vi "BT_to_neon.vi"() -> ()   [LabVIEW 2016]
uses:
  Typedef/Type_of_message_to_MCU.ctl
  Typedef/MCU_addresses.ctl
  Typedef/Serial_config_cluster.ctl
  <vilib>/Instr/_visa.llb/VISA Configure Serial Port (Instr).vi
panel:
  out "error out":errorcluster
  in  "Cluster 2":T1={"Termination Character"=10, "End Read on"=TRUE, "VISA resource name"="COM1", "baud rate"=9600, "data bits"=8, "parity"=enum."None", "stop bits"=10, "flow control"=0, "XON"=enum."DC1", "XOFF"=enum."DC3", "End Write on"=FALSE} {"Termination Character" format="%.0x"; "flow control" items=["None"=0, "XON/XOFF"=1, "RTS/CTS"=2, "DTR/DSR"=4]; "data bits" min=5 max=8 step=1; "stop bits" items=["1.0"=10, "1.5"=15, "2.0"=20]; "baud rate" items=["75"=75, "110"=110, "134"=134, "150"=150, "300"=300, "600"=600, "1200"=1200, "1800"=1800, "2400"=2400, "4800"=4800, "7200"=7200, "9600"=9600, "14400"=14400, "19200"=19200, "28800"=28800, "38400"=38400, "56000"=56000, "57600"=57600, "115200"=115200, "128000"=128000, "230400"=230400]}
  in  "Stop\n 2":bool
  in  "Read Count 2":u32=1000
  out "String 2":string
  out "Extracted Numbers 2":dbl[](array[numeric]) format="%#.6g"
  in  "Save 2":bool=TRUE
  out "Array 2":dbl[](array[numeric])
  out "Waveform Chart 2":dynamicdata(graph)
  in  "index 6":i32
  in  "index 5":i32
  in  "index 4":i32
  in  "y 2":dbl=15.0 format="%#_13g"
  in  "FIltering 2":bool
  out "Byte array has been sent 2":u8[](array[numeric])
  in  "MCU Address to be sent 2":T2
  in  "Payload  Byte to be sent 2":u8[](array[numeric])
  in  "Types of Data 2":T3
  in  "Read 2":bool=TRUE
  out "Bytes at Serial Port 2":u32
  out "error out 3":errorcluster
  in  "MAIN STOP 2":bool
  out "MAIN STOP OUT 2":bool
  in  "sEND":bool
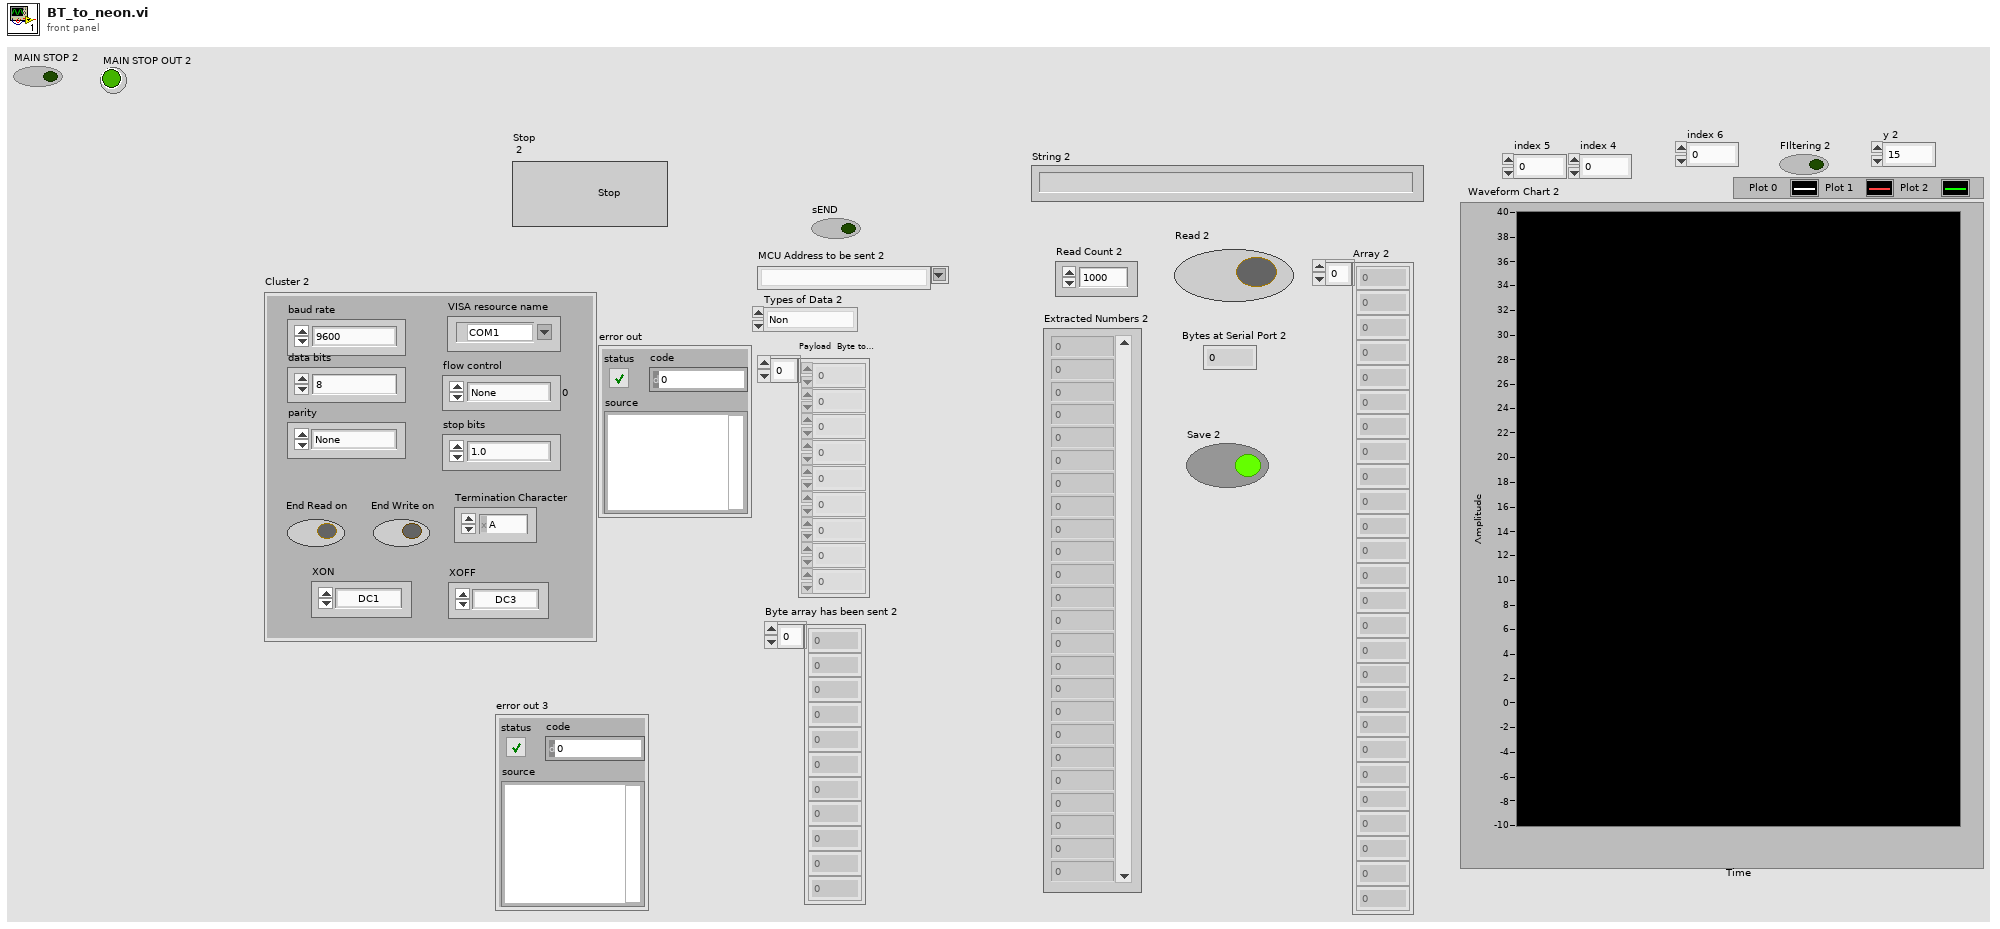
[diagram p1: front panel]
types:
  T1 = typedef "Serial_config_cluster.ctl" = cluster{"Termination Character":u8, "End Read on":bool, "VISA resource name":refnum<visa-resource-name>, "baud rate":u32, "data bits":u16, "parity":enum16{"None", "Odd", "Even", "Mark", "Space"}, "stop bits":u16, "flow control":u16, "XON":enum16{"NUL", "SOH", "STX", "ETX", "EOT", "ENQ", "ACK", "BEL", "BS", "HT", "LF", "VT", "FF", "CR", "SO", "SI", "DLE", "DC1", "DC2", "DC3", "DC4", "NAK", "SYN", "ETB", "CAN", "EM", "SUB", "ESC", "FS", "GS", "RS", "US", "SP", "!", "\"", "#", "$", "%", "&", "'", "(", ")", "*", "+", ",", "- (-)", ".", "/", "0", "1", "2", "3", "4", "5", "6", "7", "8", "9", ":", ";", "<", "=", ">", "?", "@", "A", "B", "C", "D", "E", "F", "G", "H", "I", "J", "K", "L", "M", "N", "O", "P", "Q", "R", "S", "T", "U", "V", "W", "X", "Y", "Z", "[", "\\", "]", "^", "_", "`", "a", "b", "c", "d", "e", "f", "g", "h", "i", "j", "k", "l", "m", "n", "o", "p", "q", "r", "s", "t", "u", "v", "w", "x", "y", "z", "{", "|", "}", "~"}, "XOFF":enum16{"NUL", "SOH", "STX", "ETX", "EOT", "ENQ", "ACK", "BEL", "BS", "HT", "LF", "VT", "FF", "CR", "SO", "SI", "DLE", "DC1", "DC2", "DC3", "DC4", "NAK", "SYN", "ETB", "CAN", "EM", "SUB", "ESC", "FS", "GS", "RS", "US", "SP", "!", "\"", "#", "$", "%", "&", "'", "(", ")", "*", "+", ",", "- (-)", ".", "/", "0", "1", "2", "3", "4", "5", "6", "7", "8", "9", ":", ";", "<", "=", ">", "?", "@", "A", "B", "C", "D", "E", "F", "G", "H", "I", "J", "K", "L", "M", "N", "O", "P", "Q", "R", "S", "T", "U", "V", "W", "X", "Y", "Z", "[", "\\", "]", "^", "_", "`", "a", "b", "c", "d", "e", "f", "g", "h", "i", "j", "k", "l", "m", "n", "o", "p", "q", "r", "s", "t", "u", "v", "w", "x", "y", "z", "{", "|", "}", "~"}, "End Write on":bool}
  T2 = typedef "MCU_addresses.ctl" = string
  T3 = typedef "Type_of_message_to_MCU.ctl" = enum16{"Non", "Alarm", "Error", "Time and Date", "Status", "Request", "Command"}
  T4 = enum16{"NUL", "SOH", "STX", "ETX", "EOT", "ENQ", "ACK", "BEL", "BS", "HT", "LF", "VT", "FF", "CR", "SO", "SI", "DLE", "DC1", "DC2", "DC3", "DC4", "NAK", "SYN", "ETB", "CAN", "EM", "SUB", "ESC", "FS", "GS", "RS", "US", "SP", "!", "\"", "#", "$", "%", "&", "'", "(", ")", "*", "+", ",", "- (-)", ".", "/", "0", "1", "2", "3", "4", "5", "6", "7", "8", "9", ":", ";", "<", "=", ">", "?", "@", "A", "B", "C", "D", "E", "F", "G", "H", "I", "J", "K", "L", "M", "N", "O", "P", "Q", "R", "S", "T", "U", "V", "W", "X", "Y", "Z", "[", "\\", "]", "^", "_", "`", "a", "b", "c", "d", "e", "f", "g", "h", "i", "j", "k", "l", "m", "n", "o", "p", "q", "r", "s", "t", "u", "v", "w", "x", "y", "z", "{", "|", "}", "~"}
  T5 = typedef "Message_info.ctl" = enum16{"Non", "Earthquake", "Fire", "Lost Power", "New", "Restarted"}
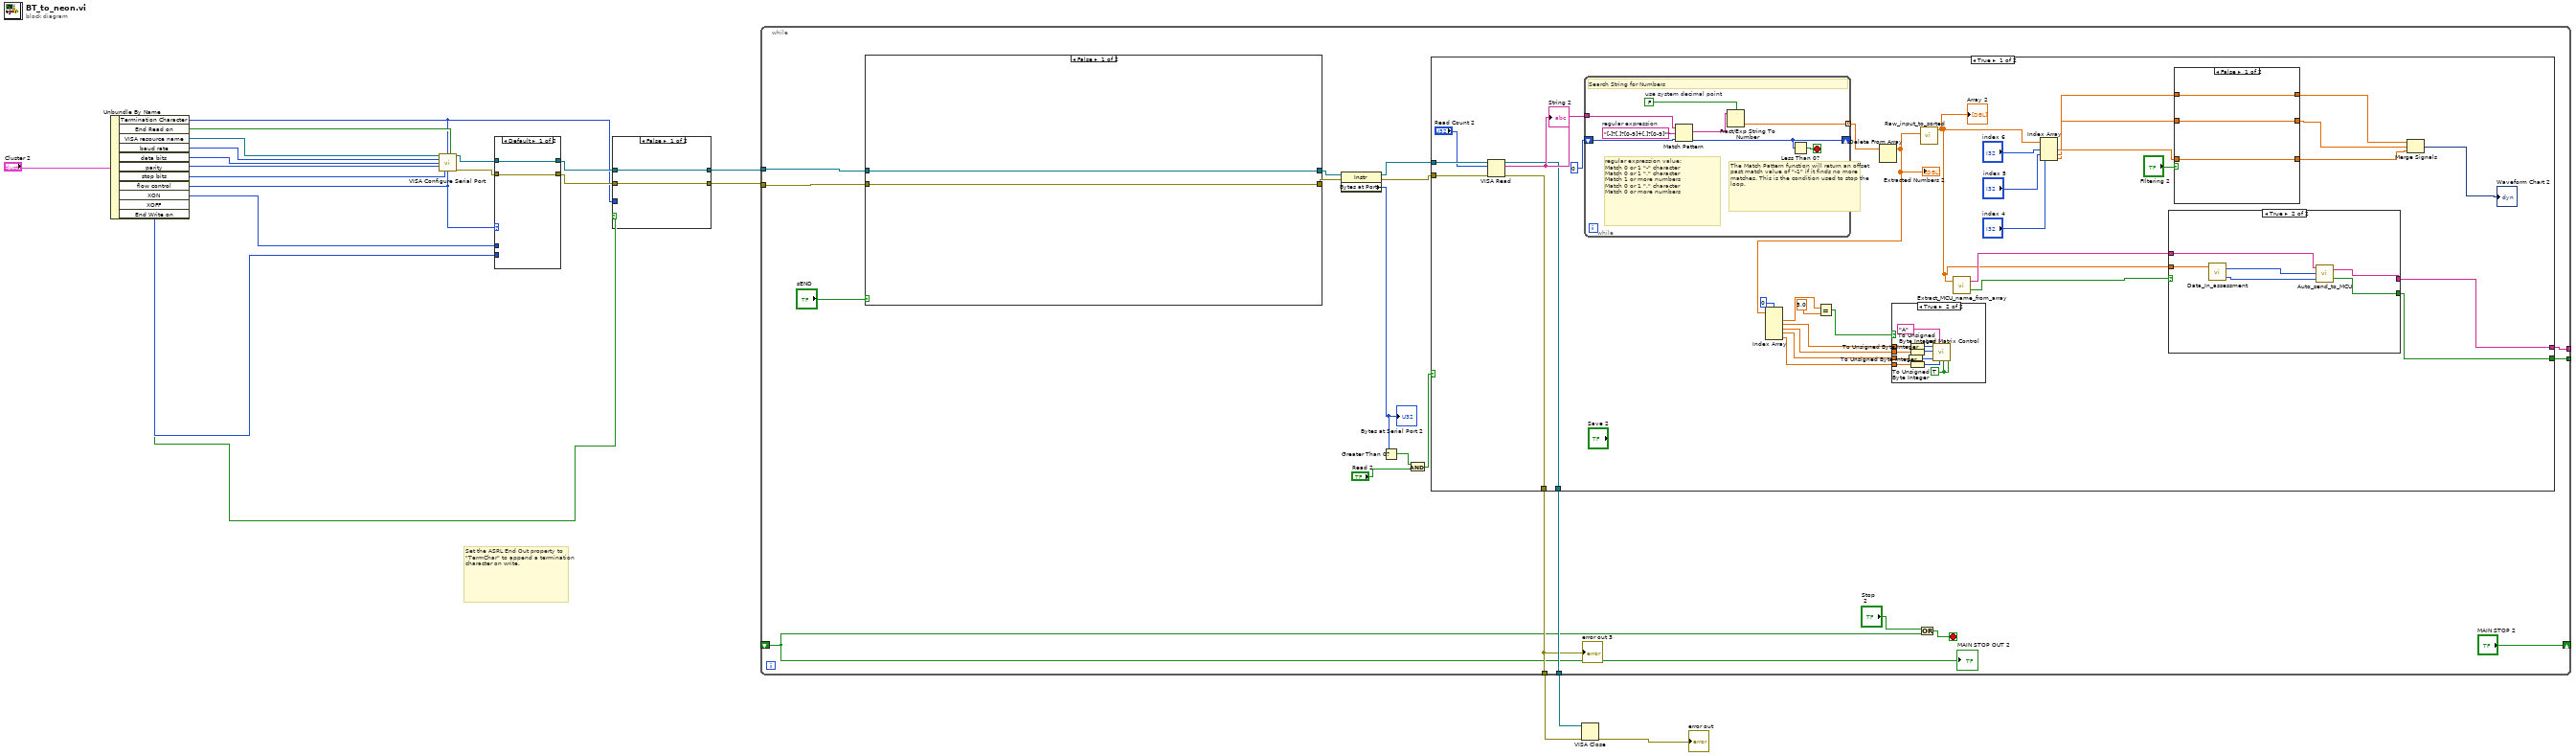
[diagram p0: block diagram]
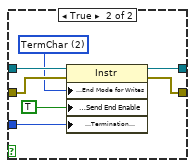
[diagram p2: hidden frame]
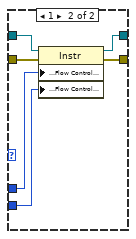
[diagram p3: hidden frame]
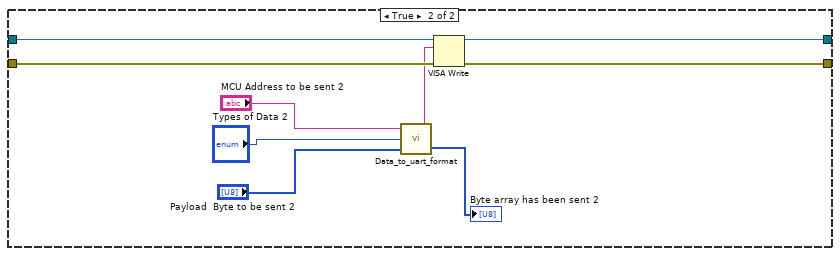
[diagram p4: hidden frame]
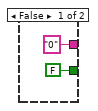
[diagram p6: hidden frame]
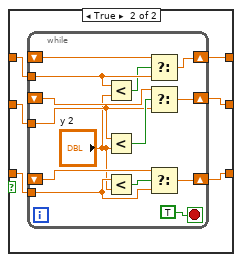
[diagram p7: hidden frame]
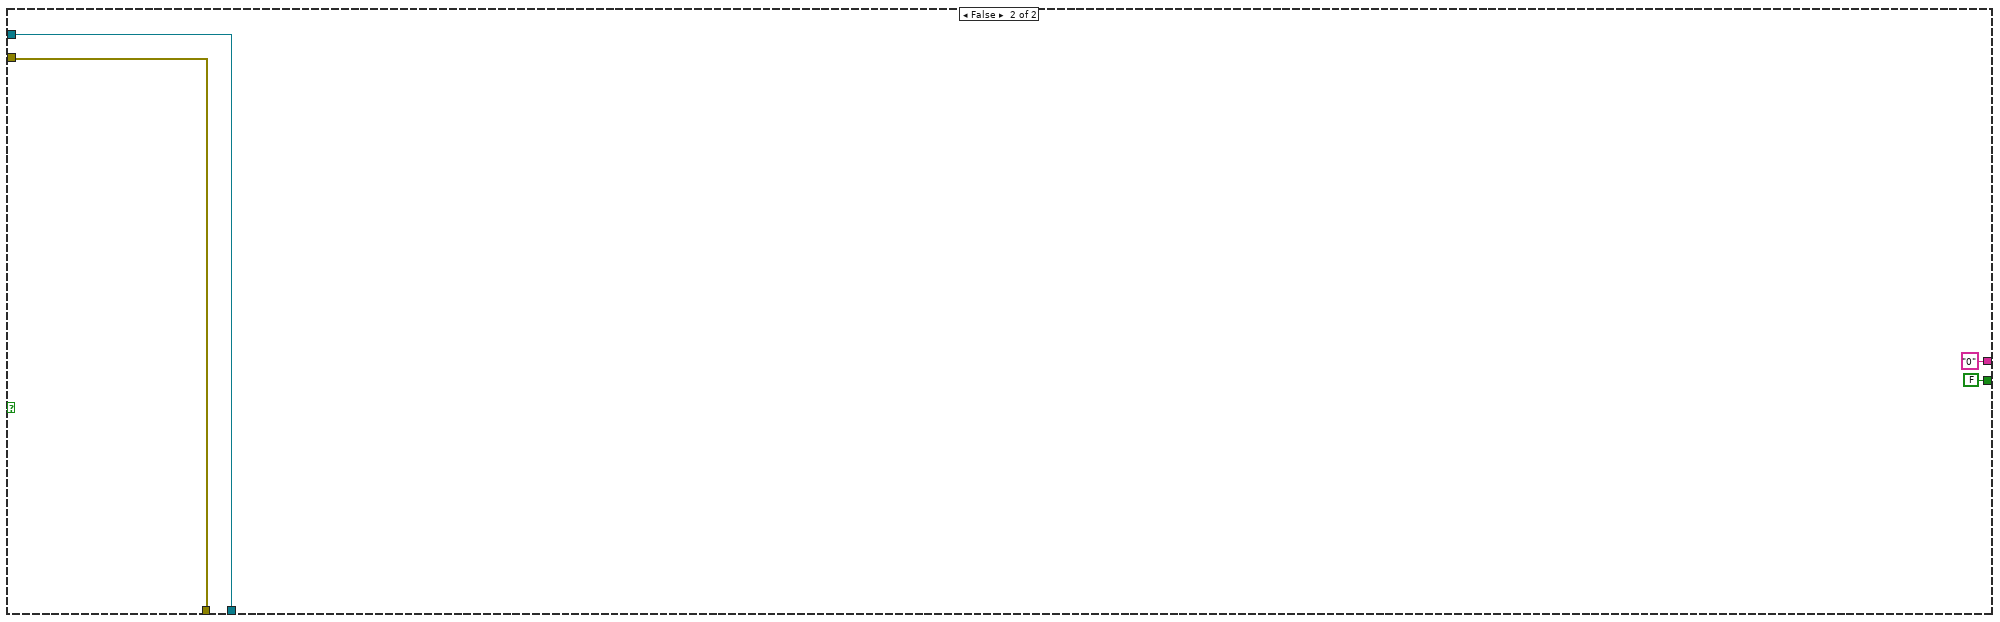
[diagram p8: hidden frame]
diagram:
  # "Set the ASRL End Out property to \"TermChar\" to append a termination character on write."
  n1 = Unbundle By Name("Cluster 2") -> ("Termination Character"=w6:u8, "End Read on"=w15:bool, "VISA resource name"=w16:refnum<visa-resource-name>, "baud rate"=w14:u32, "data bits"=w13:u16, "parity"=w12:enum16{"None", "Odd", "Even", "Mark", "Space"}, "stop bits"=w11:u16, "flow control"=w10:u16, "XON"=w9:T4, "XOFF"=w8:T4, "End Write on"=w7:bool)
  n2 = call-poly "VISA Configure Serial Port"("VISA resource name"=w16, "termination char\n(0xA = '\\n' = LF)"=w6, "Enable Termination\nChar (T)"=w15, "baud rate (9600)"=w14, "data bits (8)"=w13, "parity (0:none)"=w12, "stop bits (10: 1 bit)"=w11, "flow control (0:none)"=w10) -> ("VISA resource name out"=w19:refnum<visa-resource-name>, "error out"=w18:errorcluster)  [unwired: 2 in, 4 out]
  n3 = case shown="Default" w10 {
    tunnel: [w22 w29] -> w20
    tunnel: [w23 w28] -> w21
    tunnel: w18 -> [w22 w27]
    tunnel: w19 -> [w23 w26]
    tunnel: w9 -> [_ w25]
    tunnel: w8 -> [_ w24]
    frame Default {
    }
    frame 1 {
      n4 = property class="Instr"(reference=w26, error in=w27, "Serial Settings:Flow Control XON Character"=w25, "Serial Settings:Flow Control XOFF Character"=w24) -> (reference out=w28:refnum<visa-resource-name>, error out=w29:errorcluster)
    }
  }
  n5 = case shown="False" w7 {
    tunnel: w21 -> [w30 w38]
    tunnel: w20 -> [w31 w37]
    tunnel: [w30 w36] -> w5
    tunnel: [w31 w35] -> w4
    tunnel: w6 -> [_ w33]
    frame False {
    }
    frame True {
      w34 = u16 2 items=["None", "LastBit", "TermChar", "Break"] ("Serial Settings:Serial End Mode for Writes")
      n6 = property class="Instr"(reference=w38, error in=w37, "Serial Settings:End Mode for Writes"=w34, "Message Based Settings:Send End Enable"=TRUE, "Message Based Settings:Termination Character"=w33) -> (reference out=w36:refnum<visa-resource-name>, error out=w35:errorcluster)
    }
  }
  n7 = while {
    tunnel: w5 -> [w50]
    tunnel: w4 -> [w49]
    tunnel: [w47] -> w3
    tunnel: [w46] -> w2
    shift-right: ["MAIN STOP 2"] -> _
    shift-left: _ -> [w42]
    tunnel: [w40] -> _
    tunnel: [w39] -> _
    stop <- w44 stop-if-true
    n8 = case shown="False" "sEND" {
      tunnel: w50 -> [w59 w68]
      tunnel: w49 -> [w58 w67]
      tunnel: [w59 w66] -> w51
      tunnel: [w58 w65] -> w53
      frame False {
      }
      frame True {
        n9 = call "Data_to_uart_format.vi"("Payload  Byte to be sent"="Payload  Byte to be sent 2", "Types of Data"="Types of Data 2", "MCU Address to be sent"="MCU Address to be sent 2") -> ("Byte array has been sent"=→"Byte array has been sent 2":u8[], "Converted Message"=w61:string)
        n10 = VISA Write(VISA resource name=w68, write buffer=w61, error in (no error)=w67) -> (VISA resource name out=w66:refnum<visa-resource-name>, error out=w65:errorcluster)  [unwired: 1 out]
      }
    }
    n11 = property class="Instr"(reference=w51, error in=w53) -> (reference out=w52:refnum<visa-resource-name>, error out=w54:errorcluster, "Bytes at Port"=w55:u32)
    "Bytes at Serial Port 2" <- w55
    n12 = Greater Than 0?(x=w55) -> (x > 0?=w57:bool)
    n13 = And(x=w57, y="Read 2") -> (x .and. y?=w48:bool)
    n14 = case shown="True" w48 {
      tunnel: w52 -> [w101 w154]
      tunnel: w54 -> [w100 w153]
      tunnel: [w96 w154] -> w47
      tunnel: [w95 w153] -> w46
      tunnel: [w83 "0" ("Converted Message")] -> w40
      tunnel: [w82 FALSE ("Send/notsend")] -> w39
      frame True {
        n15 = VISA Read(VISA resource name=w101, byte count="Read Count 2", error in (no error)=w100) -> (VISA resource name out=w96:refnum<visa-resource-name>, read buffer=w97:string, error out=w95:errorcluster)  [unwired: 1 out]
        "String 2" <- w97
        n16 = while {
          tunnel: w97 -> [w150]
          shift-left: 0 -> [w148]
          shift-right: [w145] -> _
          tunnel: [w143] -> w77 mode=indexing
          stop <- w149 stop-if-true
          w147 = FALSE  # use system decimal point
          w144 = "[-]?[.]?[0-9]+[.]?[0-9]*"  # regular expression
          # "The Match Pattern function will return an offset past match value of \"-1\" if it finds no more matches. This is the condition used to stop the loop."
          # "regular expression value:\nMatch 0 or 1 \"-\" character\nMatch 0 or 1 \".\" character\nMatch 1 or more numbers\nMatch 0 or 1 \".\" character\nMatch 0 or more numbers"
          # "Search String for Numbers"
          n17 = Match Pattern(string=w150, regular expression=w144, offset (0)=w148) -> (match substring=w146:string, offset past match=w145:i32)  [unwired: 2 out]
          n18 = Fract/Exp String To Number(use system decimal point (T)=w147, string=w146) -> (number=w143:dbl)  [unwired: 2 in, 1 out]
          n19 = Less Than 0?(x=w145) -> (x < 0?=w149:bool)
        }
        n20 = Delete From Array(array=w77) -> (array with subset deleted=w69:dbl[])  [unwired: 2 in, 1 out]
        "Extracted Numbers 2" <- w69
        n21 = Index Array(array=w69, index #1=0 ("length")) -> (element #1=w75:dbl, element #2=w73:dbl, element #3=w72:dbl, element #4=w71:dbl, element #5=w70:dbl)  [unwired: 4 in]
        n22 = Equal?(x=w75, y=5.0) -> (x = y?=w74:bool)
        n23 = case shown="True" w74 {
          tunnel: w73 -> [_ w110]
          tunnel: w72 -> [_ w109]
          tunnel: w71 -> [_ w108]
          tunnel: w70 -> [_ w107]
          frame False {
          }
          frame True {
            w102 = TRUE ("Close Tab")
            n24 = To Unsigned Byte Integer(number=w108) -> (unsigned 8bit integer=w104:u8)
            n25 = To Unsigned Byte Integer(number=w110) -> (unsigned 8bit integer=w106:u8)
            n26 = To Unsigned Byte Integer(number=w109) -> (unsigned 8bit integer=w105:u8)
            n27 = To Unsigned Byte Integer(number=w107) -> (unsigned 8bit integer=w103:u8)
            n28 = call "Led Matrix Control.vi"("LED Location"=w106, "MCU addresses"=T2 "A", "Red"=w105, "Green"=w104, "Blue"=w103, "Send To MCU"=w102, "Close Tab"=w102) -> ()  [unwired: 2 in, 1 out]
          }
        }
        n29 = call "Raw_input_to_sorted.vi"("Input Array"=w69) -> ("Array Out"=w79:dbl[])  [unwired: 10 in]
        "Array 2" <- w79
        n30 = call "Extract_MCU_name_from_array.vi"("Input Array"=w79) -> ("In Range?"=w81:bool, "MCU Name"=w80:string)  [unwired: 1 in]
        n31 = Index Array(array=w79, index #1="index 6", index #2="index 5", index #3="index 4") -> (element #1=w90:dbl, element #2=w89:dbl, element #3=w88:dbl)
        n32 = case shown="True" w81 {
          tunnel: w79 -> [_ w119]
          tunnel: ["0" ("Converted Message") w116] -> w83
          tunnel: [FALSE ("Send/notsend") w115] -> w82
          tunnel: w80 -> [_ w114]
          frame False {
          }
          frame True {
            n33 = call "Data_In_assessment.vi"("Array"=w119) -> ("Message Form"=w117:T5, "Types of Data"=w118:T3)  [unwired: 1 in]
            n34 = call "Auto_send_to_MCU.vi"("Message Form"=w117, "Types of Data"=w118, "MCU Name"=w114) -> ("Send/notsend"=w115:bool, "Converted Message"=w116:string)
          }
        }
        n35 = case shown="False" "FIltering 2" {
          tunnel: w90 -> [w122 w128]
          tunnel: w89 -> [w121 w127]
          tunnel: w88 -> [w120 w126]
          tunnel: [w120 w124] -> w87
          tunnel: [w121 w123] -> w86
          tunnel: [w122 w125] -> w85
          frame False {
          }
          frame True {
            n36 = while {
              tunnel: w128 -> [w140]
              tunnel: w127 -> [w137]
              tunnel: w126 -> [w134]
              shift-right: [w131] -> w124
              shift-left: _ -> [w132]
              shift-right: [w136] -> w123
              shift-left: _ -> [w135]
              shift-right: [w142] -> w125
              shift-left: _ -> [w141]
              stop <- TRUE stop-if-true
              n37 = Less?(x=w134, y="y 2") -> (x < y?=w133:bool)
              n38 = Less?(x=w137, y="y 2") -> (x < y?=w138:bool)
              n39 = Less?(x=w140, y="y 2") -> (x < y?=w139:bool)
              n40 = Select(t=w132, s=w133, f=w134) -> (s? t:f=w131:dbl)
              n41 = Select(t=w135, s=w138, f=w137) -> (s? t:f=w136:dbl)
              n42 = Select(t=w141, s=w139, f=w140) -> (s? t:f=w142:dbl)
            }
          }
        }
        n43 = Merge Signals(w87, w86, w85) -> (→"Waveform Chart 2":dynamicdata)
      }
      frame False {
      }
    }
    "error out 3" <- w46
    n44 = Or(x="Stop\n 2", y=w42) -> (x .or. y?=w44:bool)
    "MAIN STOP OUT 2" <- w42
  }
  n45 = VISA Close(VISA resource name=w3, error in (no error)=w2) -> (error out=→"error out":errorcluster)
